vi "Multiple ERD Read & Compare To Limit.vi"(0 "GEA2 Reference In":refnum<k24>, 1 "Stand Alone":bool, 2 "Timeout":dbl, 5 "GEA Inputs":T3={"Source"=228, "Destination"=35} {"Destination" format="%.0x"; "Source" format="%.0x"}, 7 "Read ERD List":T1[](array[typedef]) {"ERD Number" format="%.0x"}, 9 "Expected Value":dbl, 11 "Error In":errorcluster, 12 "Tolerance (%)":i8=5 min=0 max=100 step=1, 13 "ERD Multiplier":dbl=1.0 format="%#_13g") -> (3 "Last value":dbl, 4 "GEA2 Reference Out":refnum<k24>, 6 "Pass/Fail?":bool, 8 "Report Text":string, 15 "Error Out":errorcluster)   [LabVIEW 2016, in "2015 VA Washer.lvlib"]
uses:
  Projects/2015 VA Washer.lvlib
  C:/Automation/DLLs/PC Dot Net/GeaCommunication.dll
  Common/LabVIEW GEA2 Toolkit/LabVIEW_GEA2_Toolkit.lvlibp/type defs/Source_Destination.ctl
  Common/LabVIEW GEA2 Toolkit/LabVIEW_GEA2_Toolkit.lvlibp/type defs/ERD Read Data In.ctl
  Common/LabVIEW GEA2 Toolkit/LabVIEW_GEA2_Toolkit.lvlibp/type defs/Data Type.ctl
  Common/LabVIEW GEA2 Toolkit/LabVIEW_GEA2_Toolkit.lvlibp
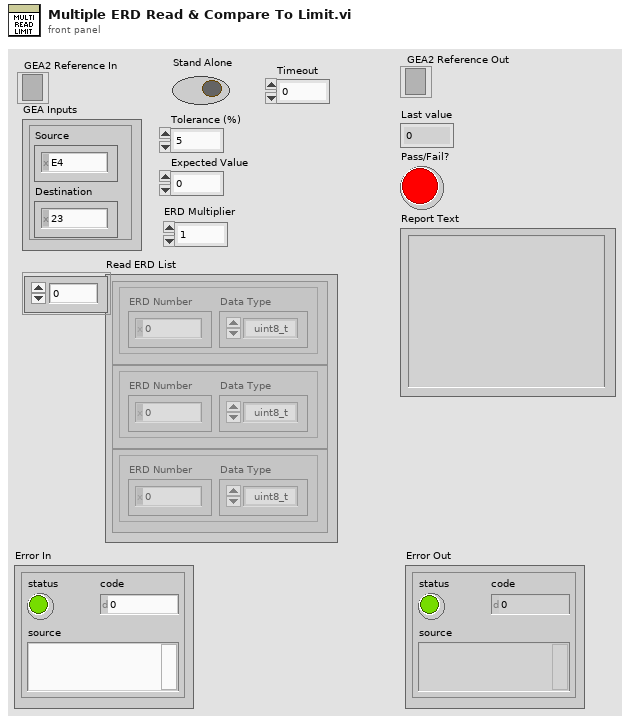
[diagram p1: front panel]
types:
  T1 = typedef "LabVIEW_GEA2_Toolkit.lvlibp/ERD Read Data In.ctl" = cluster{"ERD Number":u16, "Data Type":T2}
  T2 = typedef "LabVIEW_GEA2_Toolkit.lvlibp/Data Type.ctl" = enum16{"string", "boolean", "uint8_t", "uint16_t", "uint32_t", "uint64_t", "int8_t", "int16_t", "int32_t", "int64_t"}
  T3 = typedef "LabVIEW_GEA2_Toolkit.lvlibp/Source_Destination.ctl" = cluster{"Source":u8, "Destination":u8}
  T4 = typedef "LabVIEW_GEA2_Toolkit.lvlibp/ERD Read Data Out.ctl" = cluster{"ERD Number":u16, "Data":string}
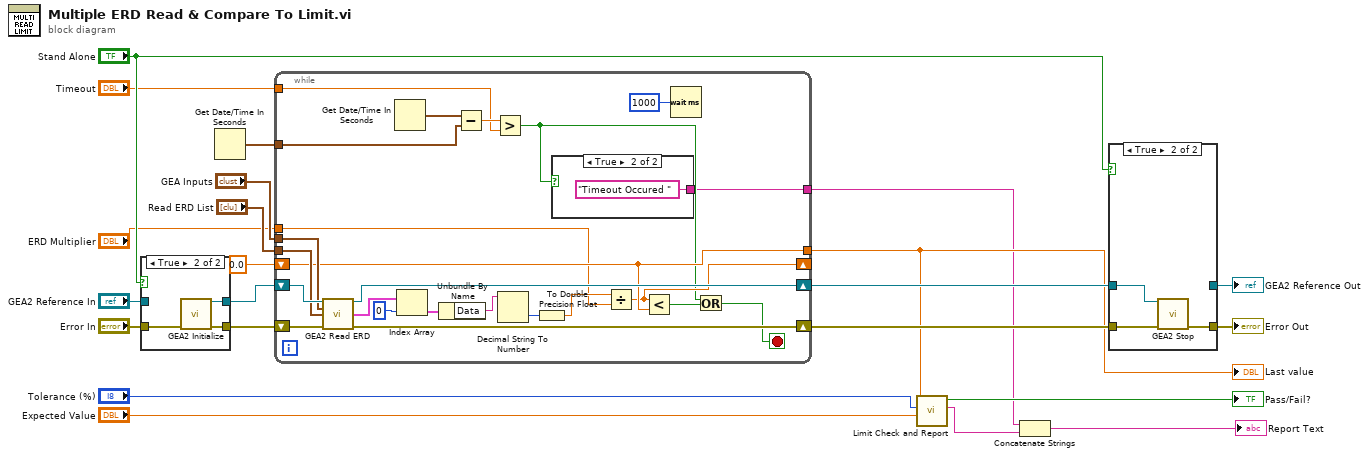
[diagram p0: block diagram]
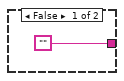
[diagram p2: hidden frame]
diagram:
  n1 = case shown="True" "Stand Alone" {
    tunnel: [w23 w27] -> w22
    tunnel: "Error In" -> [w24 w26]
    tunnel: [w24 w25] -> w18
    tunnel: "GEA2 Reference In" -> [w23 _]
    frame False {
    }
    frame True {
      n2 = call "GEA2 Initialize.vi"("error in"=w26) -> ("GEA2 Reference Out"=w27:refnum<k24>, "error out"=w25:errorcluster)  [unwired: 12 in, 1 out]
    }
  }
  n3 = Get Date/Time In Seconds() -> (seconds since 1Jan1904=w5:timestamp)
  n4 = while {
    tunnel: "GEA Inputs" -> [w47]
    tunnel: "Read ERD List" -> [w46]
    shift-right: [w50] -> w21
    shift-left: w22 -> [w51]
    shift-right: [w48] -> w17
    shift-left: w18 -> [w49]
    shift-right: [w37] -> _
    shift-left: 0.0 -> [w40]
    tunnel: [w40] -> w7
    tunnel: "ERD Multiplier" -> [w36]
    tunnel: w5 -> [w34]
    tunnel: "Timeout" -> [w32]
    tunnel: [w28] -> w3
    stop <- w30 stop-if-true
    n5 = call "GEA2 Read ERD.vi"("GEA2 Reference In"=w51, "GEA Inputs"=w47, "Read ERD List"=w46, "Error In"=w49) -> ("GEA2 Reference Out"=w50:refnum<k24>, "ERD Data Out"=w45:T4[], "Error Out"=w48:errorcluster)  [unwired: 8 in, 1 out]
    n6 = Get Date/Time In Seconds() -> (seconds since 1Jan1904=w35:timestamp)
    n7 = Index Array(array=w45, index=0) -> (element=w43:T4)
    n8 = Unbundle By Name(w43) -> ("Data"=w42:string)
    n9 = Subtract(x=w35, y=w34) -> (x-y=w33:dbl)
    n10 = Greater?(x=w33, y=w32) -> (0:w29:bool)
    n11 = Decimal String To Number(string=w42) -> (number=w39:i32)  [unwired: 2 in, 1 out]
    n12 = To Double Precision Float(number=w39) -> (double precision float=w38:dbl)
    n13 = case shown="True" w29 {
      tunnel: ["" "Timeout Occured "] -> w28
      frame False {
      }
      frame True {
      }
    }
    n14 = Divide(x=w38, y=w36) -> (x/y=w37:dbl)
    n15 = Less?(x=w37, y=w40) -> (x < y?=w31:bool)
    n16 = Wait (ms)(milliseconds to wait=u32 1000) -> ()  [unwired: 1 out]
    n17 = Or(x=w29, y=w31) -> (x .or. y?=w30:bool)
  }
  "Last value" <- w7
  n18 = call "Limit Check and Report.vi"("Expected Value"="Expected Value", "Tolerance (%)"="Tolerance (%)", "Last Value"=w7) -> ("Report Text"=w2:string, "Boolean"=→"Pass/Fail?":bool)  [unwired: 7 in]
  n19 = Concatenate Strings(w3, w2) -> (→"Report Text":string)
  n20 = case shown="True" "Stand Alone" {
    tunnel: w21 -> [w55 w58]
    tunnel: [w54 w57] -> w19
    tunnel: w17 -> [w54 w56]
    tunnel: [w55 _] -> w14
    frame False {
    }
    frame True {
      n21 = call "GEA2 Stop.vi"("GEA2 Reference In"=w58, "Error In"=w56) -> ("Error Out"=w57:errorcluster)  [unwired: 13 in]
    }
  }
  "Error Out" <- w19
  "GEA2 Reference Out" <- w14
